vi "LJM_GetHandleInfo.vi"(8 "error in":errorcluster, 11 "Handle In":i32) -> (0 "error out":errorcluster, 1 "ConnectionType":i32, 2 "DeviceType":i32, 3 "Handle Out":i32, 4 "SerialNumber":i32, 5 "Port":i32, 6 "MaxBytesPerPacket":i32, 7 "IPAddress":i32)   [LabVIEW 2022 SP3]
uses:
  labjackm.dll
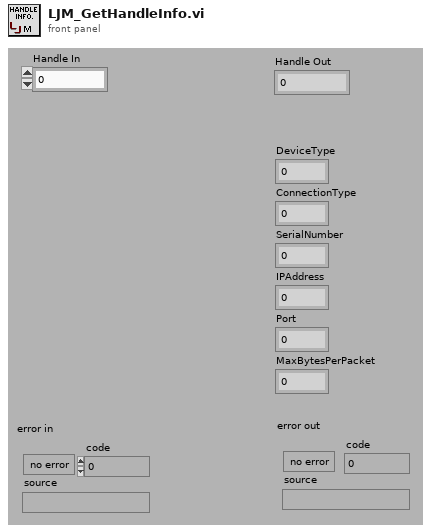
[diagram p1: front panel]
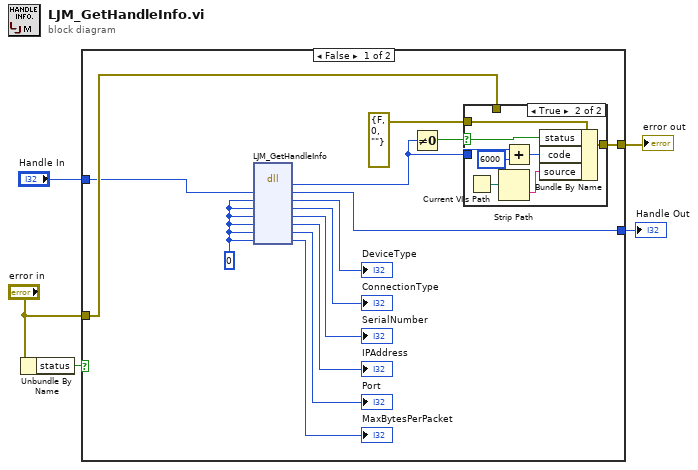
[diagram p0: block diagram]
diagram:
  n1 = Unbundle By Name("error in") -> ("status"=w4:bool)
  n2 = case shown="False" w4 {
    tunnel: [w17 w30] -> w5
    tunnel: "error in" -> [w16 w30]
    tunnel: [w7 w29] -> w2
    tunnel: "Handle In" -> [w6 w29]
    frame False {
      w9 = 0 ("Handle")
      n3 = dll-call lib="labjackm.dll" fn="LJM_GetHandleInfo"("Handle"=w6, "DeviceType"=w9, "ConnectionType"=w9, "SerialNumber"=w9, "IPAddress"=w9, "Port"=w9, "MaxBytesPerPacket"=w9) -> (w8:i32, "Handle"=w7:i32, "DeviceType"=→"DeviceType":i32, "ConnectionType"=→"ConnectionType":i32, "SerialNumber"=→"SerialNumber":i32, "IPAddress"=→"IPAddress":i32, "Port"=→"Port":i32, "MaxBytesPerPacket"=→"MaxBytesPerPacket":i32)  [unwired: 3 in, 2 out]
      n4 = Not Equal To 0?(x=w8) -> (x != 0?=w18:bool)
      n5 = case shown="True" w18 {
        selector: w18 -> [_ w27]
        tunnel: [w20 w28] -> w17
        tunnel: errorcluster {"status"=FALSE, "code"=0, "source"=""} ("error IO") -> [_ w26]
        tunnel: w8 -> [_ w22]
        tunnel: w16 -> [w20 _]
        frame False {
        }
        frame True {
          n6 = Current VI's Path() -> (path=w24:path)
          n7 = Strip Path(path=w24) -> (name=w25:string)  [unwired: 1 out]
          n8 = Add(x=w22, y=6000) -> (x+y=w23:i32)
          n9 = Bundle By Name(cluster=w26, "status"=w27, "code"=w23, "source"=w25) -> (w28:errorcluster)
        }
      }
    }
    frame True {
    }
  }
  "error out" <- w5
  "Handle Out" <- w2
